vi "Test Port Writting.vi"(8 "error in (no error)":errorcluster, 11 "TestCase in":refnum<class "LecturaADC.lvclass">) -> (0 "error out":errorcluster, 3 "TestCase out":refnum<class "LecturaADC.lvclass">)   [LabVIEW 2020]
uses:
  <vilib>/addons/_JKI Toolkits/VI Tester/TestCase.llb/TestCase.lvclass
  Simulated Device/Simulated Device.lvclass
  Cypress CY8CKIT-059/Cypress CY8CKIT-059.lvclass
  LecturaADC.lvclass
  C:/Program Files (x86)/National Instruments/LabVIEW 2020/vi.lib/addons/_JKI Toolkits/VI Tester/TestCase.llb/TestCase.lvclass
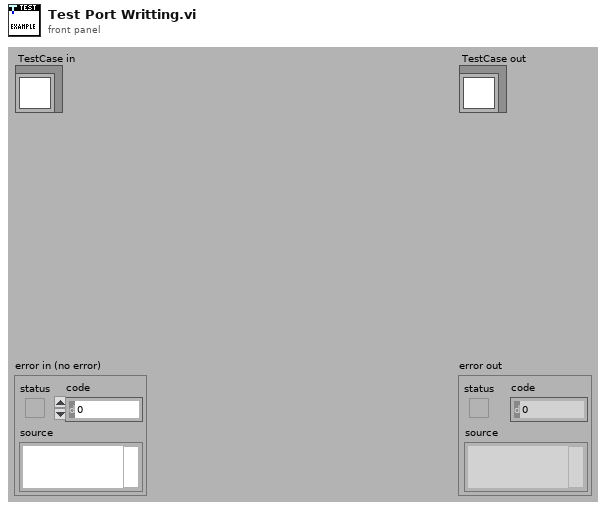
[diagram p1: front panel]
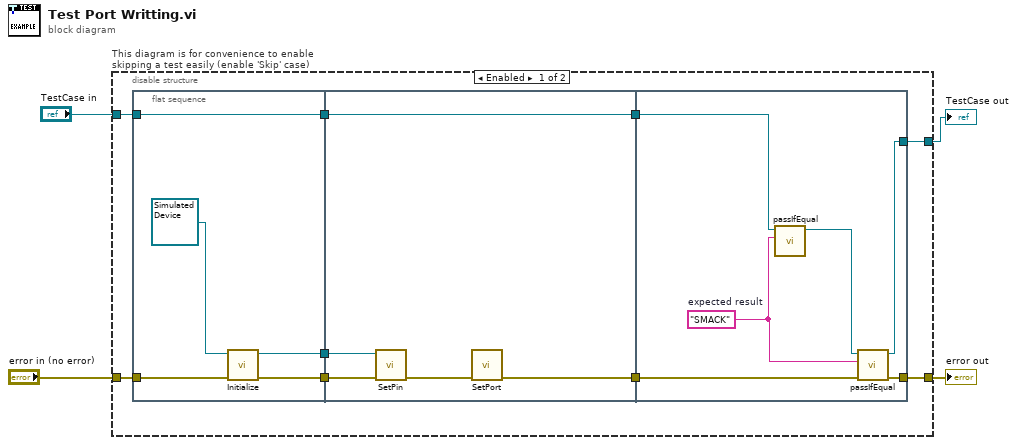
[diagram p0: block diagram]
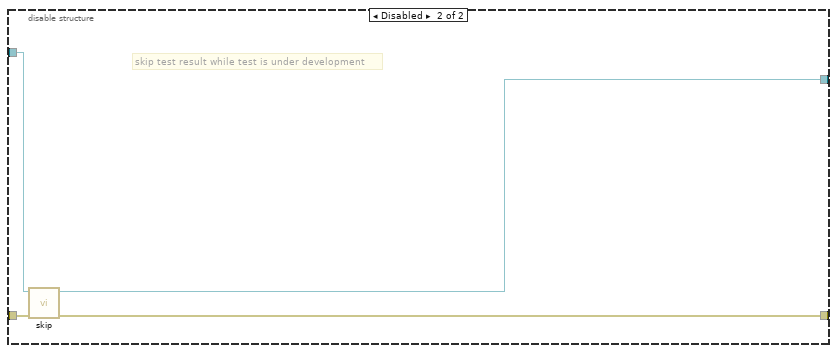
[diagram p2: hidden frame]
diagram:
  n1 = disable-structure "This diagram is for convenience to enable skipping a test easily (enable 'Skip' case)" shown="Enabled" {
    disable-tunnel: "TestCase in" -> [w13 w33]
    disable-tunnel: [w10 w31] -> w1
    disable-tunnel: [w11 w32] -> w3
    disable-tunnel: "error in (no error)" -> [w12 w30]
    frame Enabled {
      n2 = flat-sequence {
        tunnel: w13 -> [w18]
        tunnel: w12 -> [w16]
        tunnel: [w18] -> w9
        tunnel: [w15] -> w7
        tunnel: [w14] -> w5
        tunnel: w9 -> [w23]
        tunnel: [w23] -> w8
        tunnel: w7 -> [w22]
        tunnel: [w20] -> w6
        tunnel: w5 -> [w19]
        tunnel: [w29] -> w11
        tunnel: [w28] -> w10
        tunnel: w8 -> [w25]
        tunnel: w6 -> [w27]
        frame #0 {
          n3 = call-dynamic "Initialize.vi"("error in (no error)"=w16, "Simulated Device in"=refnum<class "Simulated Device.lvclass"> refnum ("Simulated Device.lvclass")) -> ("error out"=w15:errorcluster, "Simulated Device out"=w14:refnum<class "Simulated Device.lvclass">)  [unwired: 7 in, 1 out]
        }
        frame #1 {
          n4 = call-dynamic "SetPin.vi"("Simulated Device in"=w19, "error in (no error)"=w22) -> ("error out"=w21:errorcluster)  [unwired: 12 in, 1 out]
          n5 = call-dynamic "SetPort.vi"("error in (no error)"=w21) -> ("error out"=w20:errorcluster)  [unwired: 9 in, 1 out]
        }
        frame #2 {
          w24 = "SMACK"  # expected result
          n6 = call-dynamic "passIfEqual.vi"("x"=w24, "TestCase in"=w25) -> ("TestCase out"=w26:refnum<class "LecturaADC.lvclass">)  [unwired: 8 in, 1 out]
          n7 = call-dynamic "passIfEqual.vi"("error in (no error)"=w27, "x"=w24, "TestCase in"=w26) -> ("error out"=w29:errorcluster, "TestCase out"=w28:refnum<class "LecturaADC.lvclass">)  [unwired: 7 in]
        }
      }
    }
    frame Disabled {
      # "skip test result while test is under development"
      n8 = call <vilib>:"skip.vi"("error in (no error)"=w30, "TestCase in"=w33) -> ("error out"=w32:errorcluster, "TestCase out"=w31:refnum<class "LecturaADC.lvclass">)  [unwired: 8 in]
    }
  }
  "error out" <- w3
  "TestCase out" <- w1
